vi "统计亮度在一定范围内像素点个数.vi"(10 "亮度区间":cluster{"上限":i32, "下限":i32}, 11 "Histogram (端子弹片正反1)":u32[][](array[numeric])) -> (3 "数值":i32)   [LabVIEW 2014]
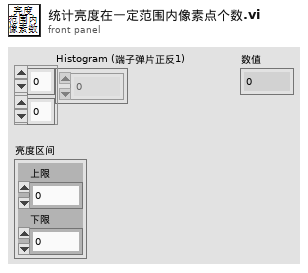
[diagram p1: front panel]
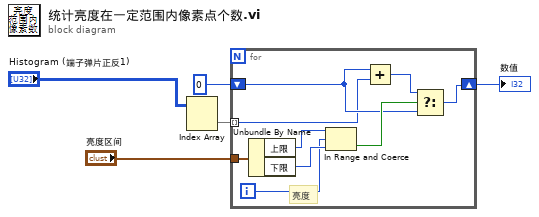
[diagram p0: block diagram]
diagram:
  n1 = Index Array(array="Histogram (端子弹片正反1)") -> (element=w2:u32[])  [unwired: 2 in]
  n2 = for {
    tunnel: w2 -> [w7] mode=indexing
    tunnel: "亮度区间" -> [w14]
    shift-right: [w10] -> w5
    shift-left: 0 -> [w8]
    i -> [w9]
    # "亮度"
    n3 = Unbundle By Name(w14) -> ("上限"=w13:i32, "下限"=w12:i32)
    n4 = In Range and Coerce(upper limit=w13, x=w9, lower limit=w12) -> (In Range?=w11:bool)  [unwired: 1 out]
    n5 = Add(x=w8, y=w7) -> (x+y=w6:u32)
    n6 = Select(t=w6, s=w11, f=w8) -> (s? t:f=w10:u32)
  }
  "数值" <- w5
